vi "Wait for NIT.vi"(8 "Error":errorcluster, 10 "NIT Start":u32, 11 "session in":refnum<k21>) -> (0 "Error out":errorcluster, 3 "session out":refnum<k21>)   [LabVIEW 2010, in "XNET Reflective Memory Custom Device.lvlib"]
uses:
  XNET Reflective Memory Custom Device.lvlib
  <vilib>/xnet/xnet.llb/XNET Read (State FlexRay Cycle Macrotick).vi
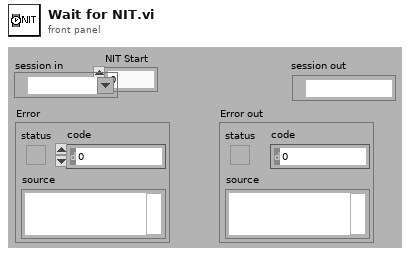
[diagram p1: front panel]
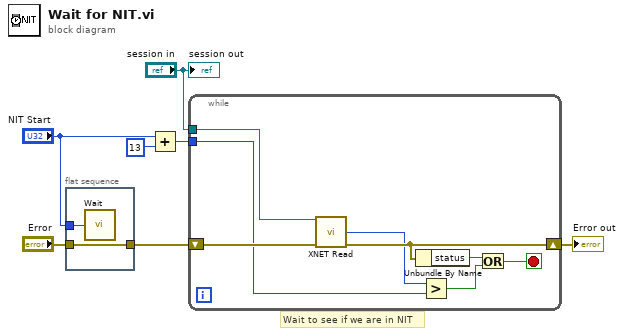
[diagram p0: block diagram]
diagram:
  # "Wait to see if we are in NIT"
  n1 = flat-sequence {
    tunnel: [w9] -> w6
    tunnel: "Error" -> [w9]
    tunnel: "NIT Start" -> [w8]
    frame #0 {
      n2 = call "Wait"("Count(uSec)"=w8) -> ()  [unwired: 1 out]
    }
  }
  n3 = Add(x="NIT Start", y=u32 13) -> (x+y=w3:u32)
  n4 = while {
    tunnel: "session in" -> [w17]
    shift-right: [w12] -> w4
    shift-left: w6 -> [w16]
    tunnel: w3 -> [w15]
    stop <- w11 stop-if-true
    n5 = call-poly <vilib>:"XNET Read.vi"("session in"=w17, "error in (no error)"=w16) -> ("macrotick"=w10:u16, "error out"=w12:errorcluster)  [unwired: 10 in, 2 out]
    n6 = Unbundle By Name(w12) -> ("status"=w13:bool)
    n7 = Greater?(x=w10, y=w15) -> (0:w14:bool)
    n8 = Or(x=w13, y=w14) -> (x .or. y?=w11:bool)
  }
  "Error out" <- w4
  "session out" <- "session in"
